vi "Current Conumption Test.vi"(8 "error in":errorcluster, 10 "LED INI":T1 {"Settings"."Source V" format="%#_g V"; "Settings"."VLED 3" format="%#_g V"; "Settings"."VLED 2" format="%#_g V"; "Settings"."VLED 1" format="%#f V"; "Limits"."Wavelength" format="%#_g nm"; "Limits"."Tolerance" format="%#_g %"; "Limits"."Current 3" format="%#_g  mA"; "Limits"."Current 2" format="%#_g  mA"; "Limits"."Current 1" format="%#_g mA"; "Instruments"."Resistor 3" format="%#_g ohm"; "Instruments"."Resistor 2" format="%#_g ohm"; "Instruments"."Resistor 1" format="%#f ohm"}, 11 "Test Visualize In":refnum<vi>) -> (0 "error out":errorcluster, 2 "Pass Fail":bool, 3 "Test Visualize Out":refnum<vi>)   [LabVIEW 2018, in "LED Control Module.lvlib"]
uses:
  LED Control Module.lvlib
  INI/INI File Control.ctl
  Public Controls/LVS Testplan.ctl
  Public Controls/LVS Instruments.ctl
  Public Controls/LVS Limits.ctl
  Public Controls/LVS Settings.ctl
  <vilib>/Analysis/6fits.llb/Curve Fitting Criteria.ctl
  <vilib>/Analysis/6fits.llb/General Linear Fit Algorithm.ctl
  <userlib>/_OpenG.lib/numeric/numeric.llb/Random Number Within Range - DBL__ogtk.vi
  <vilib>/Analysis/polynomials.llb/1D Polynomial Evaluation (DBL).vi
  <vilib>/Analysis/NI_AALPro.lvlib
  INI/LED INI File.lvlib
panel:
  out "Array 3":bool[](array[boolean])
  out "Test Visualize":cluster{dbl[], dbl[]}[](graph)=[{[0.0, 0.0, 0.0], [0.0, nan, nan]}, {[-0.05, 0.0], [0.0, 0.0]}, {[-0.05, 0.0], [0.0, 0.0]}] caption="LED Current Consumption"
  # "Data Input"
  # "Local data"
  # "Data Output"
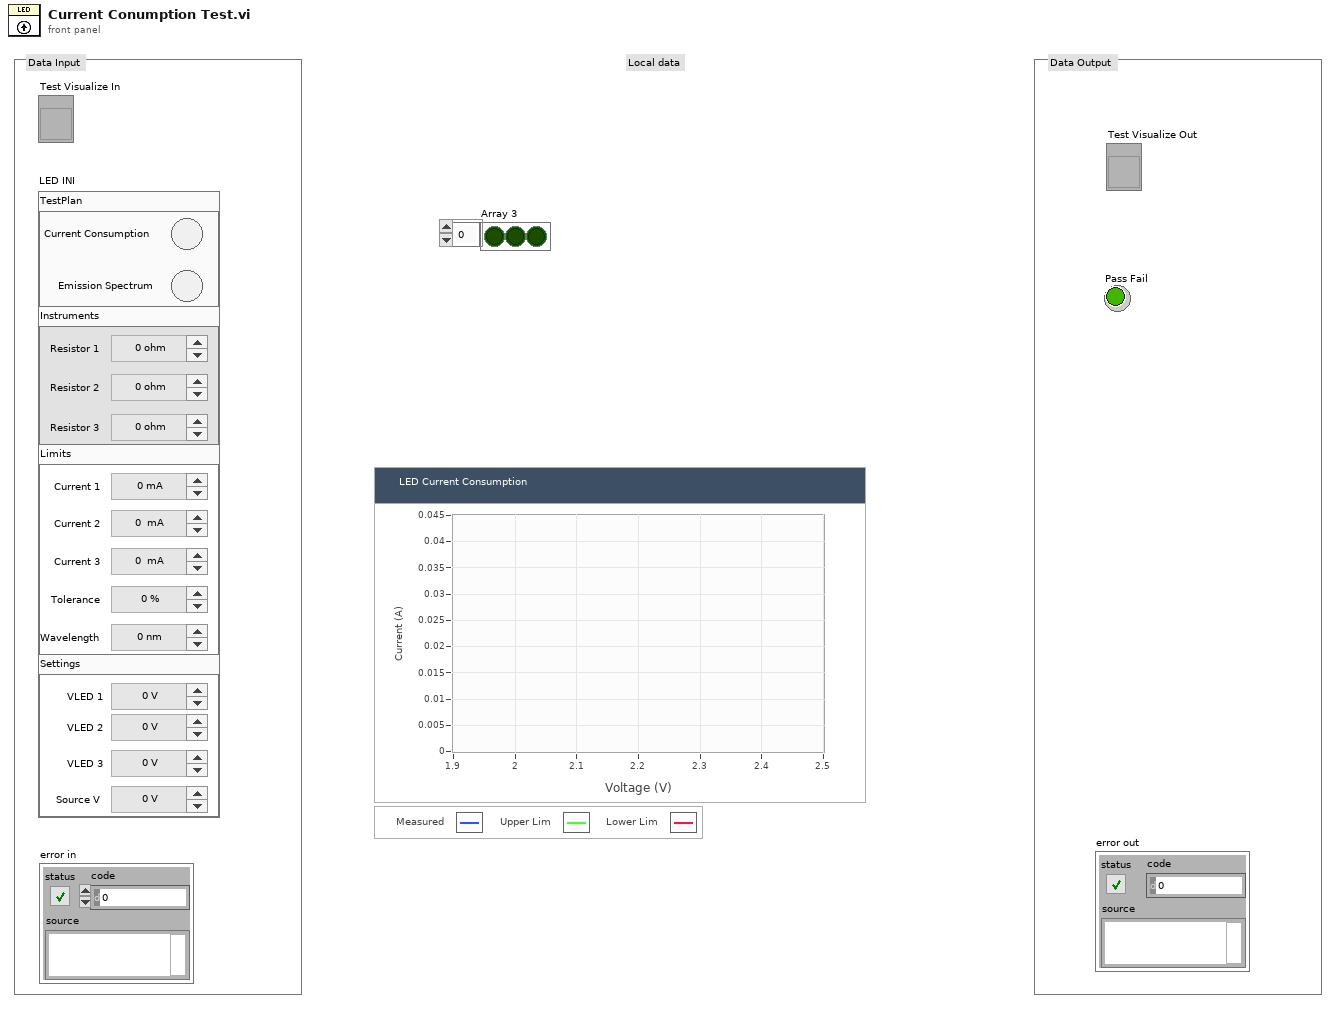
[diagram p1: front panel]
types:
  T1 = typedef "LED Control Module.lvlib/LED INI File.lvlib/INI File Control.ctl" = cluster{"TestPlan":T2, "Instruments":T3, "Limits":T4, "Settings":T5}
  T2 = typedef "LED Control Module.lvlib/LVS Testplan.ctl" = cluster{"Current Consumption":bool, "Emission Spectrum":bool}
  T3 = typedef "LED Control Module.lvlib/LVS Instruments.ctl" = cluster{"Resistor 1":dbl, "Resistor 2":dbl, "Resistor 3":dbl}
  T4 = typedef "LED Control Module.lvlib/LVS Limits.ctl" = cluster{"Current 1":dbl, "Current 2":dbl, "Current 3":dbl, "Tolerance":dbl, "Wavelength":dbl}
  T5 = typedef "LED Control Module.lvlib/LVS Settings.ctl" = cluster{"VLED 1":dbl, "VLED 2":dbl, "VLED 3":dbl, "Source V":dbl}
  T6 = cluster{"X Scale.Name Label.Text":string, "Y Scale.Name Label.Text":string, "Label.Text":string}
  T7 = typedef "NI_AALPro.lvlib/General Linear Fit Algorithm.ctl" = u16
  T8 = typedef "NI_AALPro.lvlib/Curve Fitting Criteria.ctl" = u16
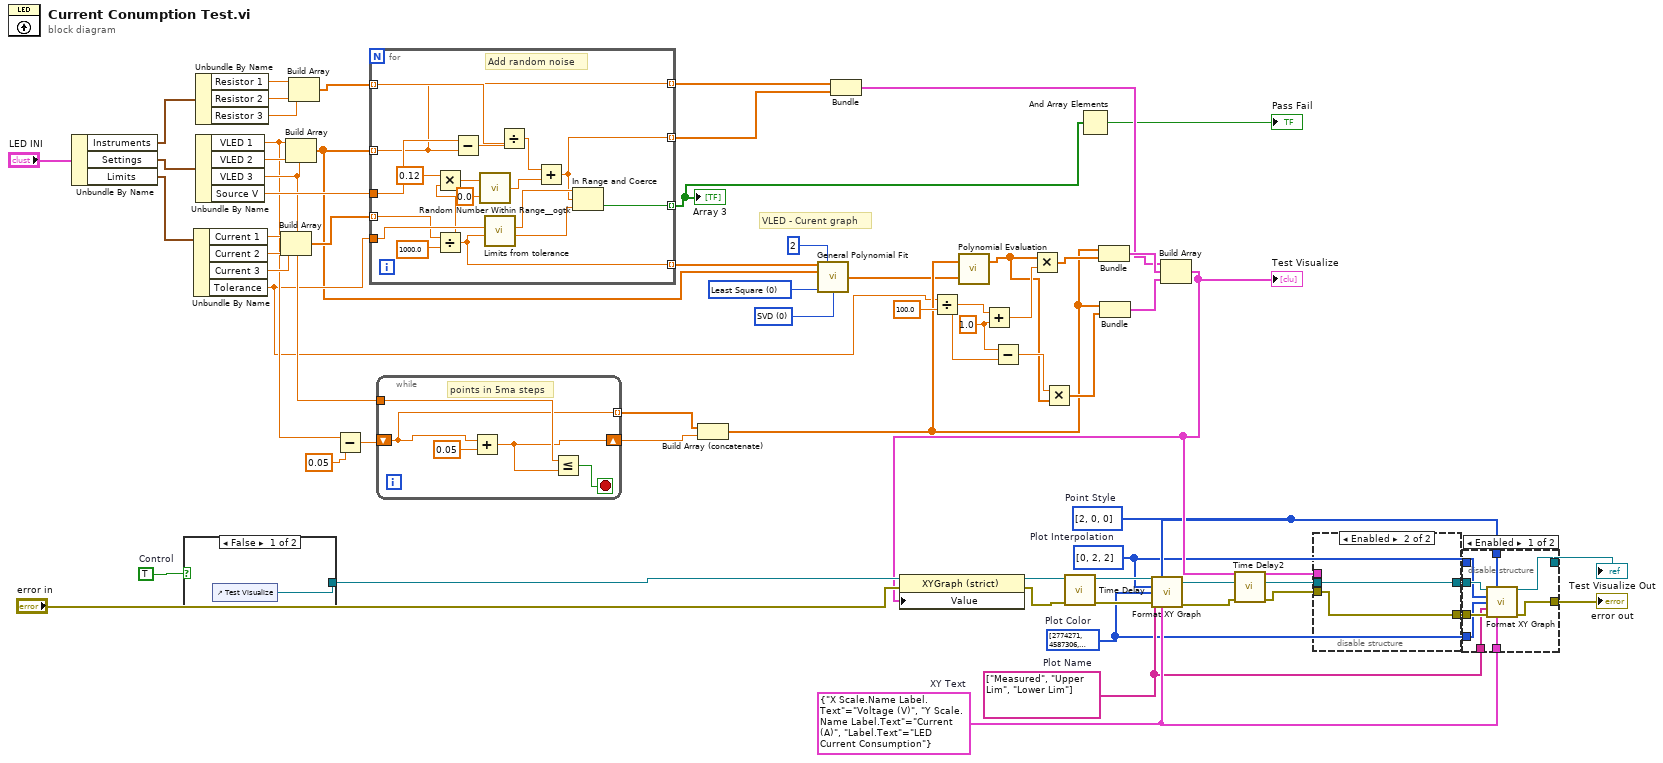
[diagram p0: block diagram]
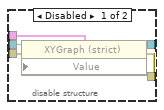
[diagram p2: hidden frame]
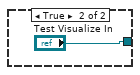
[diagram p4: hidden frame]
diagram:
  w9 = T6 {"X Scale.Name Label.Text"="Voltage (V)", "Y Scale.Name Label.Text"="Current (A)", "Label.Text"="LED Current Consumption"}  # XY Text
  w33 = TRUE  # Control
  w8 = string[] ["Measured", "Upper Lim", "Lower Lim"]  # Plot Name
  w3 = u32[] [2774271, 4587306, 16716354, 65351, 5898088, 3731200]  # Plot Color
  w4 = u8[] [0, 2, 2]  # Plot Interpolation
  w7 = u8[] [2, 0, 0]  # Point Style
  w51 = 1.0 ("y")
  w29 = T7 0 items=["SVD", "Givens", "Givens2", "Householder", "LU Decomposition", "Cholesky", "SVD for Rank Deficient H"] ("algorithm")
  w30 = T8 0 items=["Least Square", "Least Absolute Residual", "Bisquare"] ("method")
  # "VLED - Curent graph"
  n1 = Unbundle By Name("LED INI") -> ("Instruments"=w21:T3, "Settings"=w20:T5, "Limits"=w19:T4)
  n2 = case shown="False" w33 {
    tunnel: [w63 "Test Visualize In"] -> w18
    frame False {
      n3 = control-ref of="Test Visualize"() -> (w63:refnum<vi>)
    }
    frame True {
    }
  }
  n4 = Unbundle By Name(w19) -> ("Current 1"=w58:dbl, "Current 2"=w57:dbl, "Current 3"=w56:dbl, "Tolerance"=w32:dbl)
  n5 = Unbundle By Name(w21) -> ("Resistor 1"=w62:dbl, "Resistor 2"=w61:dbl, "Resistor 3"=w60:dbl)
  n6 = Unbundle By Name(w20) -> ("VLED 1"=w37:dbl, "VLED 2"=w59:dbl, "VLED 3"=w53:dbl, "Source V"=w54:dbl)
  n7 = Build Array(w58, w57, w56) -> (w31:dbl[])
  n8 = Build Array(w37, w59, w53) -> (w27:dbl[])
  n9 = Build Array(w62, w61, w60) -> (w55:dbl[])
  n10 = Subtract(x=w37, y=0.05) -> (x-y=w39:dbl)
  n11 = for {
    tunnel: w55 -> [w80] mode=indexing
    tunnel: w27 -> [w78] mode=indexing
    tunnel: w31 -> [w71] mode=indexing
    tunnel: w54 -> [w81]
    tunnel: [w66] -> w41 mode=indexing
    tunnel: [w78] -> w42 mode=indexing
    tunnel: w32 -> [w77]
    tunnel: [w75] -> w24 mode=indexing
    tunnel: [w65] -> w26 mode=indexing
    # "Add random noise"
    n12 = Divide(x=w71, y=1000.0) -> (x/y=w65:dbl)
    n13 = Multiply(x=0.12, y=w65) -> (x*y=w73:dbl)
    n14 = Subtract(x=w81, y=w78) -> (x-y=w79:dbl)
    n15 = call-poly <userlib>:"Random Number Within Range__ogtk.vi"("High"=w73, "Low"=0.0) -> ("Random Number"=w67:dbl)  [unwired: 3 in]
    n16 = call "Limits from tolerance.vi"("Nominal"=w65, "Tolerance %"=w77) -> ("Min Limit"=w69:dbl, "Max Limit"=w76:dbl)  [unwired: 8 in]
    n17 = Divide(x=w79, y=w80) -> (x/y=w68:dbl)
    n18 = Add(x=w68, y=w67) -> (x+y=w66:dbl)
    n19 = In Range and Coerce(upper limit=w76, x=w66, lower limit=w69) -> (In Range?=w75:bool)  [unwired: 1 out]
  }
  "Array 3" <- w24
  n20 = while {
    tunnel: w53 -> [w85]
    shift-right: [w84] -> w36
    shift-left: w39 -> [w82]
    tunnel: [w82] -> w35 mode=indexing
    stop <- w83 stop-if-true
    # "points in 5ma steps"
    n21 = Add(x=w82, y=0.05) -> (x+y=w84:dbl)
    n22 = Less Or Equal?(x=w85, y=w84) -> (x <= y?=w83:bool)
  }
  n23 = Build Array (concatenate)(w35, w36) -> (w34:dbl[])
  n24 = call <vilib>:"General Polynomial Fit.vi"("Y"=w26, "polynomial order"=2, "X"=w27, "method"=w30, "algorithm"=w29) -> ("Polynomial Coefficients"=w28:dbl[])  [unwired: 7 in, 3 out]
  n25 = Bundle(w42, w41) -> (w40:cluster{dbl[], dbl[]})  [unwired: 1 in]
  n26 = Divide(x=w32, y=100.0) -> (x/y=w50:dbl)
  n27 = call-poly <vilib>:"Polynomial Evaluation.vi"("P(x)"=w28, "A"=w34) -> ("P(A)"=w47:dbl[])  [unwired: 1 out]
  n28 = Add(x=w50, y=w51) -> (x+y=w49:dbl)
  n29 = Subtract(x=w51, y=w50) -> (x-y=w48:dbl)
  n30 = Multiply(x=w47, y=w49) -> (x*y=w45:dbl[])
  n31 = Multiply(x=w48, y=w47) -> (x*y=w44:dbl[])
  n32 = And Array Elements(Boolean array=w24) -> (logical AND=→"Pass Fail":bool)
  n33 = Bundle(w34, w45) -> (w43:cluster{dbl[], dbl[]})  [unwired: 1 in]
  n34 = Bundle(w34, w44) -> (w46:cluster{dbl[], dbl[]})  [unwired: 1 in]
  n35 = Build Array(w40, w43, w46) -> (w14:cluster{dbl[], dbl[]}[])
  "Test Visualize" <- w14
  n36 = property class="XYGraph (strict)"(reference=w18, error in="error in", "Value"=w14) -> (reference out=w17:refnum<vi>, error out=w13:errorcluster)
  n37 = call "Time Delay"("error in (no error)"=w13) -> ("error out"=w12:errorcluster)  [unwired: 10 in]
  n38 = call "Format XY Graph.vi"("XYGraph in"=w17, "Point Style"=w7, "Plot Interpolation"=w4, "Plot Color"=w3, "Plot Name"=w8, "error in (no error)"=w12, "XY Text"=w9) -> ("XYGraph out"=w15:refnum<vi>, "error out"=w2:errorcluster)  [unwired: 7 in]
  n39 = call "Time Delay2"("error in (no error)"=w2) -> ("error out"=w1:errorcluster)  [unwired: 10 in]
  n40 = disable-structure shown="Enabled" {
    disable-tunnel: w15 -> [w91 w92]
    disable-tunnel: w14 -> [w90 _]
    disable-tunnel: [w89 w93] -> w11
    disable-tunnel: [w88 w92] -> w6
    disable-tunnel: w1 -> [w87 w93]
    frame Disabled {
      n41 = property class="XYGraph (strict)"(reference=w91, error in=w87, "Value"=w90) -> (reference out=w88:refnum<vi>, error out=w89:errorcluster)
    }
    frame Enabled {
    }
  }
  n42 = disable-structure shown="Enabled" {
    disable-tunnel: w11 -> [w102 w103]
    disable-tunnel: [w101 w103] -> w10
    disable-tunnel: w9 -> [w100 _]
    disable-tunnel: w8 -> [w99 _]
    disable-tunnel: w7 -> [w98 _]
    disable-tunnel: w6 -> [w97 _]
    disable-tunnel: [w96 _] -> w5
    disable-tunnel: w4 -> [w95 _]
    disable-tunnel: w3 -> [w94 _]
    frame Enabled {
      n43 = call "Format XY Graph.vi"("XYGraph in"=w97, "Point Style"=w98, "Plot Interpolation"=w95, "Plot Color"=w94, "Plot Name"=w99, "error in (no error)"=w102, "XY Text"=w100) -> ("XYGraph out"=w96:refnum<vi>, "error out"=w101:errorcluster)  [unwired: 7 in]
    }
    frame Disabled {
    }
  }
  "error out" <- w10
  "Test Visualize Out" <- w5
